vi "MGI Boolean Debounce.vi"(1 "Filter Length":i32, 2 "Input":bool) -> (0 "Output":bool)   [LabVIEW 2016]
doc: "Output is true only if Input is true for the previous Filter Length calls. Reentrant.\n\nAuthored by David A. Moore\nsupport@mooregoodideas.com\nwww.mooregoodideas.com\n\nCopyright (c) 2010, Moore Good Ideas, Inc.\n\nAll rights reserved.\n\nRedistribution and use in source and binary forms, with or without modification, are permitted provided that the following conditions are met:\n\n * Redistributions of source code must retain the above copyright notice, this list of conditions and the following disclaimer.\n * Redistributions in binary form must reproduce the above copyright notice, this list of conditions and the following disclaimer in the documentation and/or other materials provided with the distribution.\n * Neither the name of Moore Good Ideas, Inc. nor the names of its contributors may be used to endorse or promote products derived from this software without specific prior written permission.\n\nTHIS SOFTWARE IS PROVIDED BY THE COPYRIGHT HOLDERS AND CONTRIBUTORS \"AS IS\" AND ANY EXPRESS OR IMPLIED WARRANTIES, INCLUDING, BUT NOT LIMITED TO, THE IMPLIED WARRANTIES OF MERCHANTABILITY AND FITNESS FOR A PARTICULAR PURPOSE ARE DISCLAIMED. IN NO EVENT SHALL THE COPYRIGHT OWNER OR CONTRIBUTORS BE LIABLE FOR ANY DIRECT, INDIRECT, INCIDENTAL, SPECIAL, EXEMPLARY, OR CONSEQUENTIAL DAMAGES (INCLUDING, BUT NOT LIMITED TO, PROCUREMENT OF SUBSTITUTE GOODS OR SERVICES; LOSS OF USE, DATA, OR PROFITS; OR BUSINESS INTERRUPTION) HOWEVER CAUSED AND ON ANY THEORY OF LIABILITY, WHETHER IN CONTRACT, STRICT LIABILITY, OR TORT (INCLUDING NEGLIGENCE OR OTHERWISE) ARISING IN ANY WAY OUT OF THE USE OF THIS SOFTWARE, EVEN IF ADVISED OF THE POSSIBILITY OF SUCH DAMAGE."
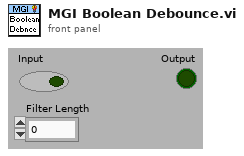
[diagram p1: front panel]
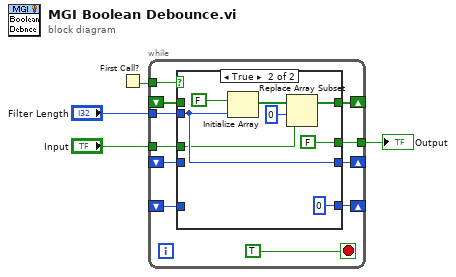
[diagram p0: block diagram]
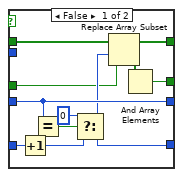
[diagram p2: hidden frame]
diagram:
  n1 = First Call?() -> (First Call?: T/F=w4:bool)
  n2 = while {
    tunnel: w4 -> [w14]
    shift-right: [w12] -> _
    shift-left: _ -> [w7]
    tunnel: "Filter Length" -> [w13]
    shift-right: [w11] -> _
    shift-left: _ -> [w8]
    shift-right: [w10] -> _
    shift-left: _ -> [w9]
    tunnel: "Input" -> [w6]
    tunnel: [w5] -> w1
    stop <- TRUE stop-if-true
    n3 = case shown="True" w14 {
      tunnel: w13 -> [_ w31]
      tunnel: [w17 w29] -> w12
      tunnel: [w23 w31] -> w11
      tunnel: [w19 0] -> w10
      tunnel: w9 -> [w25 _]
      tunnel: w8 -> [w23 _]
      tunnel: w7 -> [w20 _]
      tunnel: w6 -> [w18 w28]
      tunnel: [w16 FALSE] -> w5
      frame False {
        n4 = Increment(x=w25) -> (x+1=w22:i32)
        n5 = Equal?(x=w23, y=w22) -> (x = y?=w24:bool)
        n6 = Select(t=0, s=w24, f=w22) -> (s? t:f=w19:i32)
        n7 = Replace Array Subset(array=w20, new element=w18, index=w19) -> (w17:bool[])
        n8 = And Array Elements(Boolean array=w17) -> (logical AND=w16:bool)
      }
      frame True {
        n9 = Initialize Array(FALSE, w31) -> (w33:bool[])
        n10 = Replace Array Subset(array=w33, new element=w28, index=0) -> (w29:bool[])
      }
    }
  }
  "Output" <- w1
